vi "retrieveData.vi"(8 "error in (no error)":errorcluster, 11 "EncoderReader in":refnum<class "EncoderReader.lvclass">) -> (0 "error out":errorcluster, 3 "EncoderReader out":refnum<class "EncoderReader.lvclass">)   [LabVIEW 2013, in "EncoderReader.lvlib" / "EncoderReader.lvclass"]
uses:
  <userlib>/Common/Devices/EncoderReader/EncoderReader/EncoderReader.lvclass
  <userlib>/Common/Devices/EncoderReader/EncoderReader/EncoderReader.lvclass/EncoderReader.ctl
  <userlib>/Common/SerialProtocols/SerialCommunicator/SerialCommunicator.lvclass
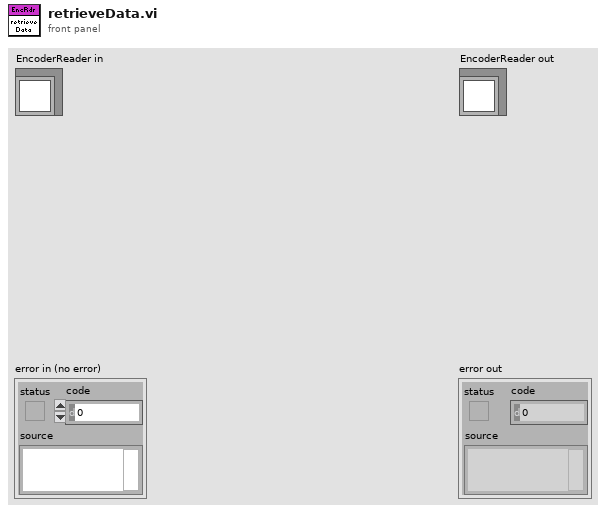
[diagram p1: front panel]
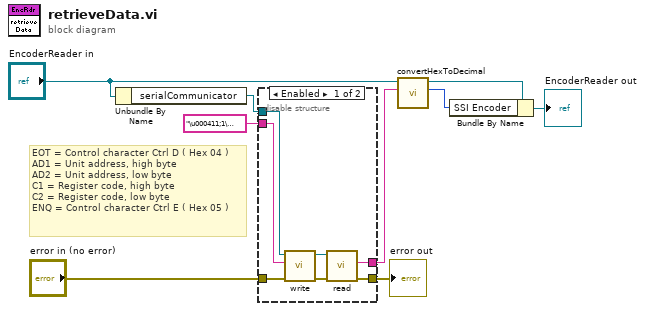
[diagram p0: block diagram]
diagram:
  # "EOT = Control character Ctrl D ( Hex 04 )\nAD1 = Unit address, high byte\nAD2 = Unit address, low byte\nC1 = Register code, high byte\nC2 = Register code, low byte\nENQ = Control character Ctrl E ( Hex 05 )"
  n1 = Unbundle By Name("EncoderReader in") -> ("serialCommunicator"=w9:refnum<class "SerialCommunicator.lvclass">)
  n2 = disable-structure shown="Enabled" {
    disable-tunnel: w9 -> [w16 _]
    disable-tunnel: "error in (no error)" -> [w15 _]
    disable-tunnel: [w14 _] -> w7
    disable-tunnel: "\u000411;1\u0005" ("Send") -> [w11 _]
    disable-tunnel: [w10 _] -> w1
    frame Enabled {
      n3 = call-dynamic "write.vi"("error in (no error)"=w15, "writeString"=w11, "SerialCommunicator in"=w16) -> ("error out"=w12:errorcluster, "SerialCommunicator out"=w13:refnum<class "SerialCommunicator.lvclass">)  [unwired: 7 in]
      n4 = call-dynamic "read.vi"("error in (no error)"=w12, "SerialCommunicator in"=w13) -> ("error out"=w14:errorcluster, "stringRead"=w10:string)  [unwired: 7 in, 1 out]
    }
    frame Disabled {
    }
  }
  "error out" <- w7
  n5 = call <userlib>:"convertHexToDecimal.vi"("hexString"=w1, "EncoderReader in"="EncoderReader in") -> ("decimalValue"=w5:i32, "EncoderReader out"=w4:refnum<class "EncoderReader.lvclass">)  [unwired: 6 in, 2 out]
  n6 = Bundle By Name(cluster=w4, "SSI Encoder"=w5) -> (→"EncoderReader out":refnum<class "EncoderReader.lvclass">)
